vi "MEMR-Get Calibration Files.vi"(0 "Params":T1, 7 "Data Folder":path, 11 "error in (no error)":errorcluster) -> (4 "Probe":path, 8 "Elicitor":path, 15 "error out":errorcluster)   [LabVIEW 2020]
uses:
  Typedefs/MEMR-Params.ctl
  Typedefs/MEMR-Probe.ctl
  Typedefs/MEMR-Elicitor.ctl
  Human Studies/SFM Frontend/LV Source/Typedefs/HSTS-Transducer.ctl
  Typedefs/MEMR-Sequence.ctl
  Typedefs/MEMR-Analysis.ctl
  Typedefs/MEMR-Timing.ctl
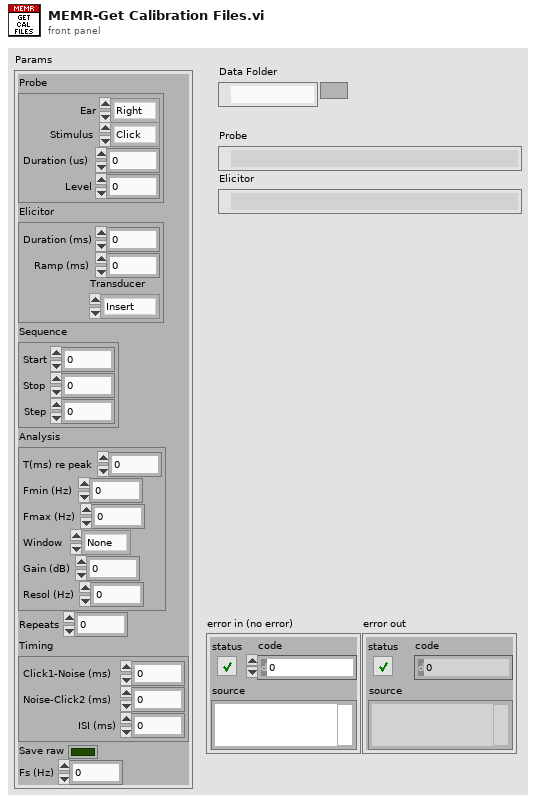
[diagram p1: front panel]
types:
  T1 = typedef "MEMR-Params.ctl" = cluster{"Probe":T2, "Elicitor":T3, "Sequence":T5, "Analysis":T6, "Repeats":i32, "Timing":T7, "Save raw":bool, "Fs (Hz)":dbl}
  T2 = typedef "MEMR-Probe.ctl" = cluster{"Ear":enum16{"Right", "Left"}, "Stimulus":enum16{"Click", "Chirp"}, "Duration (us)":dbl, "Level":dbl}
  T3 = typedef "MEMR-Elicitor.ctl" = cluster{"Duration (ms)":dbl, "Ramp (ms)":dbl, "Transducer":T4}
  T4 = typedef "HSTS-Transducer.ctl" = enum16{"Insert", "TDH-39", "HD300", "ER-10X"}
  T5 = typedef "MEMR-Sequence.ctl" = cluster{"Start":dbl, "Stop":dbl, "Step":dbl}
  T6 = typedef "MEMR-Analysis.ctl" = cluster{"T(ms) re peak":dbl, "Fmin (Hz)":dbl, "Fmax (Hz)":dbl, "Window":enum16{"None", "Hanning", "Hamming"}, "Gain (dB)":dbl, "Resol (Hz)":dbl}
  T7 = typedef "MEMR-Timing.ctl" = cluster{"Click1-Noise (ms)":dbl, "Noise-Click2 (ms)":dbl, "ISI (ms)":dbl}
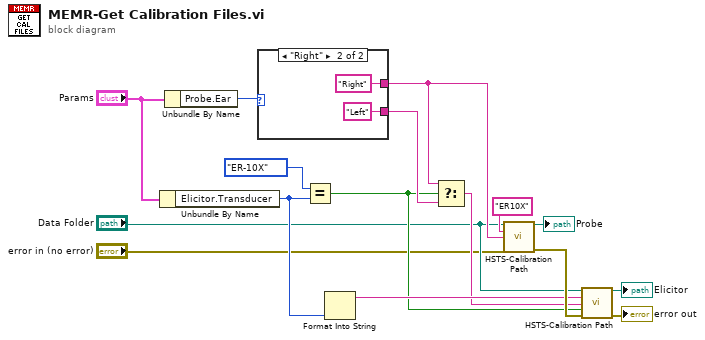
[diagram p0: block diagram]
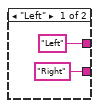
[diagram p2: hidden frame]
diagram:
  n1 = Unbundle By Name("Params") -> ("Elicitor.Transducer"=w6:T4)
  n2 = Unbundle By Name("Params") -> ("Probe.Ear"=w15:enum16{"Right", "Left"})
  n3 = case shown="\"Right\"" w15 {
    tunnel: ["Left" "Right"] -> w11
    tunnel: ["Right" "Left"] -> w10
    frame "Left" {
    }
    frame "Right" {
    }
  }
  n4 = Equal?(x=HSTS-Transducer."ER-10X" ("y"), y=w6) -> (x = y?=w7:bool)
  n5 = Format Into String(w6) -> (resulting string=w13:string)  [unwired: 3 in, 1 out]
  n6 = Select(t=w11, s=w7, f=w10) -> (s? t:f=w8:string)
  n7 = call "HSTS-Calibration Path.vi"("Data Folder"="Data Folder", "Speaker"="ER10X", "Side"=w11, "error in (no error)"="error in (no error)") -> ("Cal Path"=→"Probe":path, "error out"=w16:errorcluster)  [unwired: 10 in]
  n8 = call "HSTS-Calibration Path.vi"("Data Folder"="Data Folder", "Speaker"=w13, "Side"=w8, "Secondary"=w7, "error in (no error)"=w16) -> ("Cal Path"=→"Elicitor":path, "error out"=→"error out":errorcluster)  [unwired: 9 in]
